vi "HumanNetwork.vi"(8 "error in (no error)":errorcluster) -> (0 "error out":errorcluster)   [LabVIEW 2023]
doc: "Human Network\n\nInput\n --Error in \n\nOutput\n --Error out"
uses:
  HumanGlobal.vi
  <vilib>/Rock Robotics/Network Tables/NT Write Boolean.vi
  <vilib>/Rock Robotics/Network Tables/NT Write Number.vi
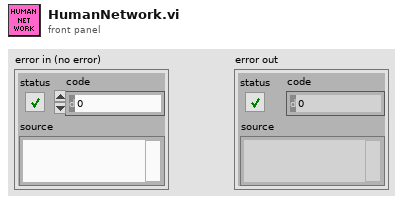
[diagram p1: front panel]
types:
  T1 = typedef "HumanDriveModeENUM.ctl" = enum16{"0 - Normal Swerve", "1 - Auto traj  - Left Speaker", "2 - Auto traj - Center Speaker", "3 - Auto traj - Speaker Right", "4 - Auto traj - Amp", "5 - Auto traj - Source", "6 - Auto traj -  Left Stage", "7 - Auto traj - Center Stage", "8 - Auto traj - Right Stage"}
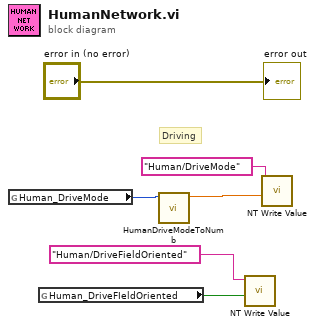
[diagram p0: block diagram]
diagram:
  # "Driving"
  n1 = global read "HumanGlobal.vi" "Human_DriveMode"() -> (w4:T1)
  n2 = global read "HumanGlobal.vi" "Human_DriveFIeldOriented"() -> (w1:bool)
  n3 = call "HumanDriveModeToNumb.vi"("Human_DriveMode"=w4) -> ("StateNumber"=w3:dbl)  [unwired: 10 in]
  n4 = call-poly <vilib>:"NT Write Value.vi"("value"=w1, "name"="Human/DriveFieldOriented") -> ()  [unwired: 9 in, 1 out]
  n5 = call-poly <vilib>:"NT Write Value.vi"("value"=w3, "name"="Human/DriveMode") -> ()  [unwired: 9 in, 1 out]
  "error out" <- "error in (no error)"
